vi "Decode Reply.vi"(5 "ProcessID":u32 format="%04x", 6 "RxTimeStamp":u32, 7 "TxTimeStamp Alt":u32, 10 "ICMP Packet Info":T3 {"Sequence Number" format="%04x"; "ID" format="%04x"; "Checksum" format="%04x"; "Data" format="%02x"}, 11 "IP Packet":T2 {"Header Checksum" format="%04x"; "Flags" format="%02x"; "Type of Service" format="%02x"}) -> (0 "Error Out":errorcluster, 1 "Done?":bool, 3 "Ping Reply Info":T1 {"Sequence" format="%04x"})   [LabVIEW 2018]
uses:
  ICMP Packet Info.ctl
  IP Packet Info.ctl
  Ping Reply Info.ctl
  Instance           2 20Saved   Decode Reply .vi
  Instance           1 20Saved   Decode Reply .vi
panel:
  in  "Error In":errorcluster
  # "Use the process ID we obtained when sending the ping to make sure we have received the correct reply"
  # "The tick count is encoded in the ping packet, but if we want to try and make\na time measurement more accurate we can use a time stamp taken when\nthe packet is sent, not when it is encoded.  This deprives us of being able\nto send a bunch of pings at the same time and calculate arrival time back,\nbut that's ok in most circumstances."
  # "U8"
  # "U8"
  # "U16"
  # "U16"
  # "U16"
  # "U32"
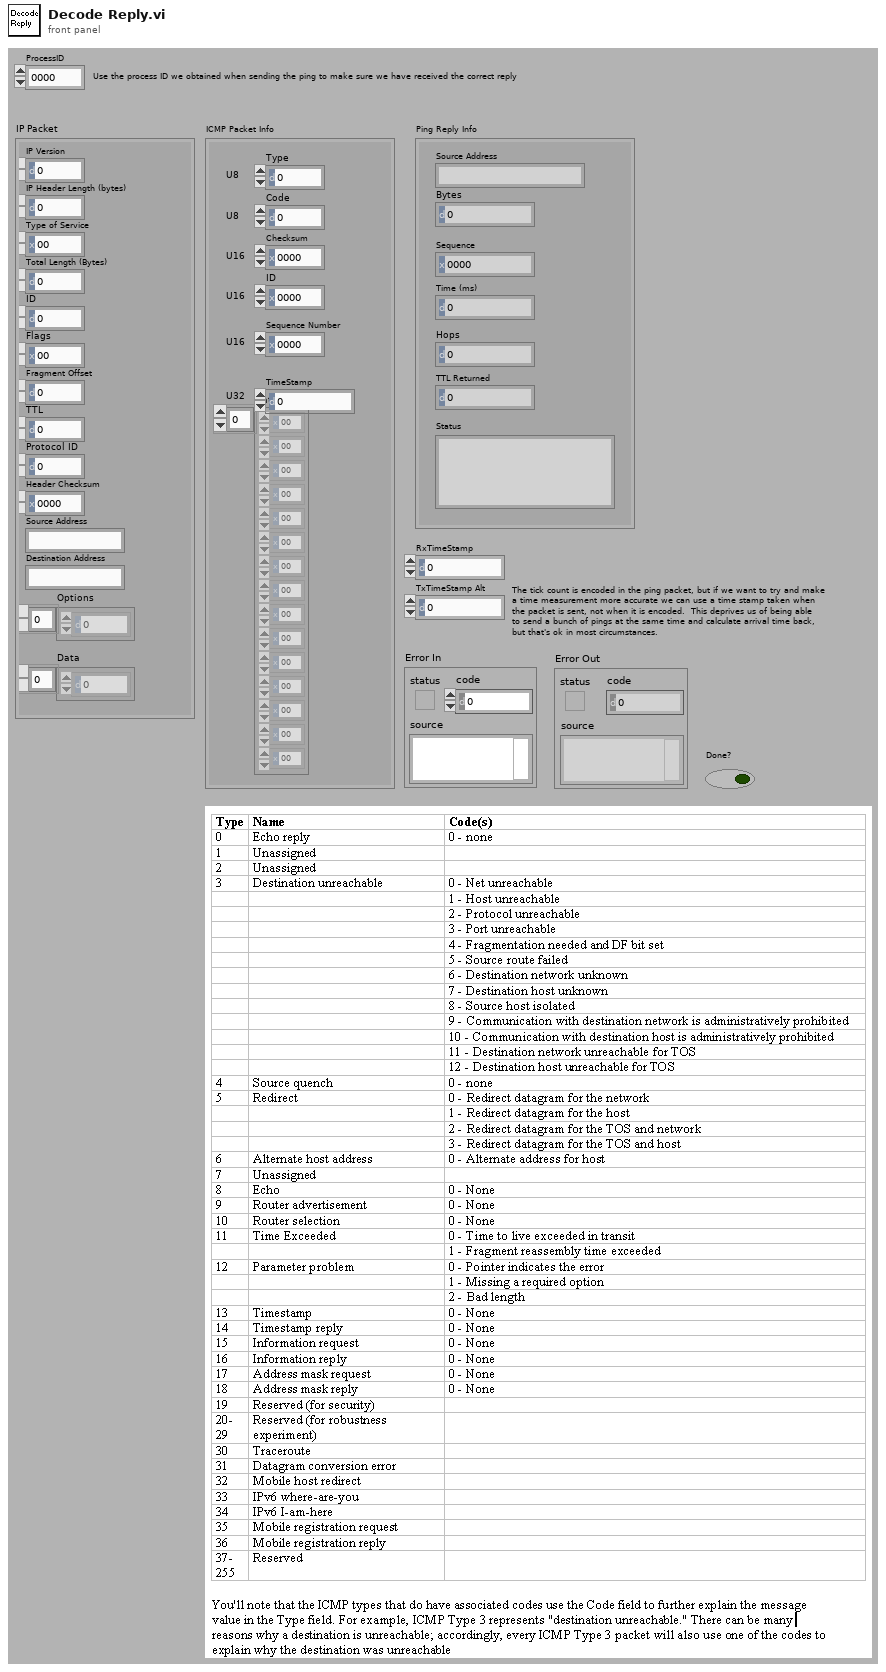
[diagram p1: front panel]
types:
  T1 = typedef "Ping Reply Info.ctl" = cluster{"Source Address":string, "Bytes":i32, "Sequence":u16, "Time (ms)":i32, "Hops":u8, "TTL Returned":u8, "Status":string}
  T2 = typedef "IP Packet Info.ctl" = cluster{"IP Version":u8, "IP Header Length (bytes)":u8, "Type of Service":u8, "ID":u16, "Flags":u8, "Total Length (Bytes)":u16, "Fragment Offset":u16, "TTL":u8, "Protocol ID":u8, "Header Checksum":u16, "Source Address":string, "Destination Address":string, "Options":u8[], "Data":u8[]}
  T3 = typedef "ICMP Packet Info.ctl" = cluster{"Type":u8, "Code":u8, "Checksum":u16, "ID":u16, "Sequence Number":u16, "TimeStamp":u32, "Data":u8[]}
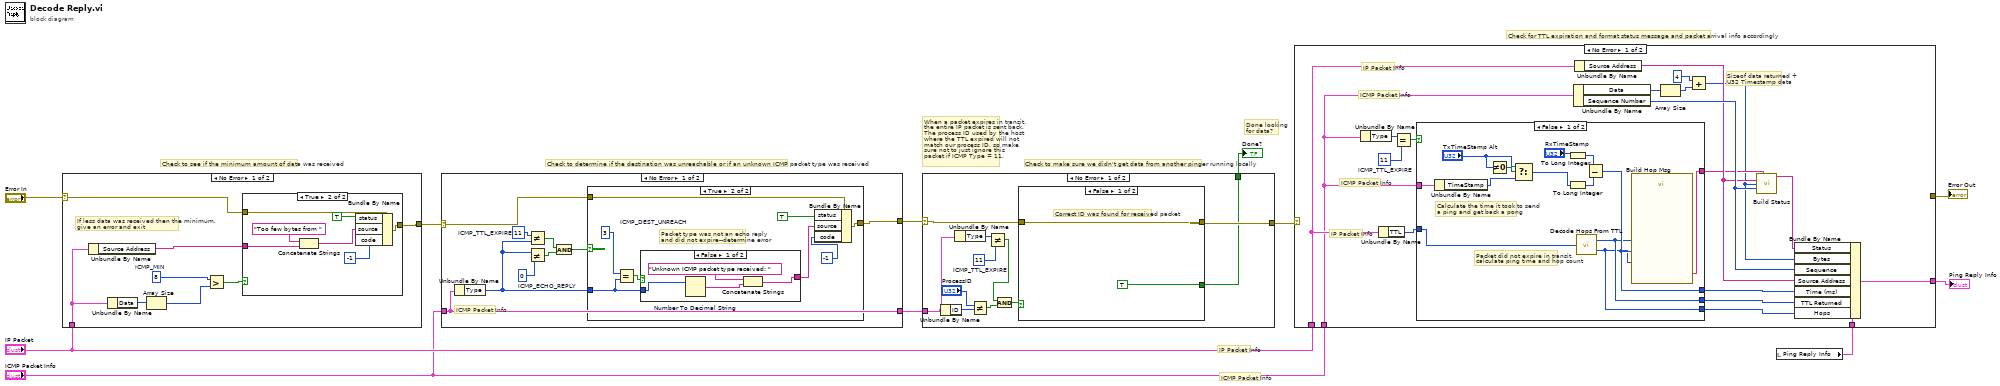
[diagram p0: block diagram]
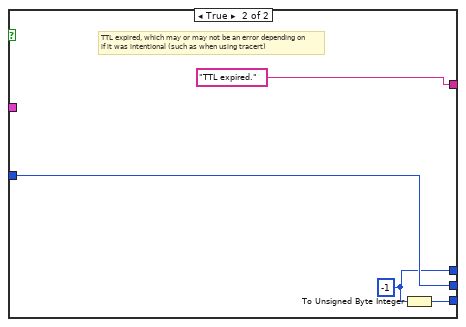
[diagram p2: hidden frame]
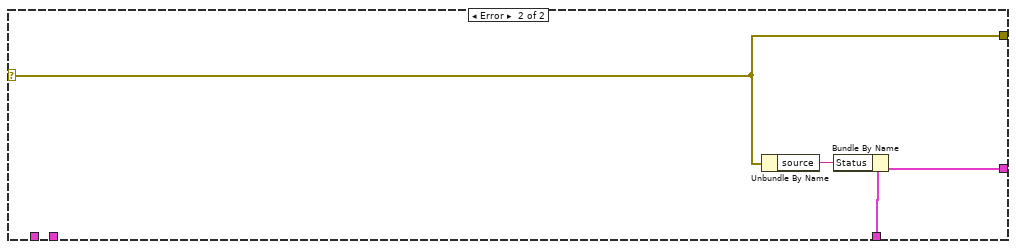
[diagram p3: hidden frame]
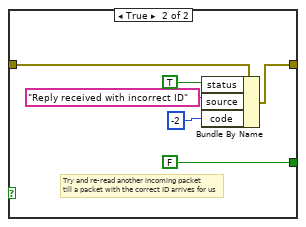
[diagram p4: hidden frame]
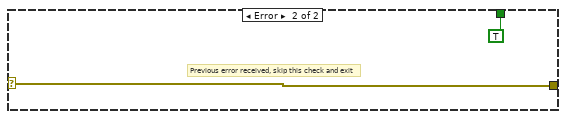
[diagram p5: hidden frame]
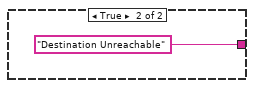
[diagram p7: hidden frame]
diagram:
  # "Done looking\nfor data?"
  # "When a packet expires in transit,\nthe entire IP packet is sent back.\nThe process ID used by the host\nwhere the TTL expired will not\nmatch our process ID, so make\nsure not to just ignore this \npacket if ICMP Type = 11."
  # "Check for TTL expiration and format status message and packet arrival info accordingly"
  # "ICMP Packet Info"
  # "IP Packet Info"
  # "Check to make sure we didn't get data from another pinger running locally"
  # "Check to determine if the destination was unreachable or if an unknown ICMP packet type was received"
  # "Check to see if the minimum amount of data was received"
  n1 = case shown="No Error" "Error In" {
    selector: "Error In" -> [w18 w28]
    tunnel: [w17 w28] -> w10
    tunnel: "IP Packet" -> [w16 _]
    frame No Error {
      w12 = u8 8  # ICMP_MIN
      # "If less data was received then the minimum,\ngive an error and exit"
      n2 = Unbundle By Name(w16) -> ("Source Address"=w19:string)
      n3 = Unbundle By Name(w16) -> ("Data"=w15:u8[])
      n4 = Array Size(array=w15) -> (size(s)=w14:i32)
      n5 = Greater?(x=w12, y=w14) -> (0:w13:bool)
      n6 = case shown="True" w13 {
        tunnel: w19 -> [_ w27]
        tunnel: w18 -> [w20 w26]
        tunnel: [w20 w23] -> w17
        frame False {
        }
        frame True {
          n7 = Concatenate Strings("Too few bytes from ", w27) -> (w25:string)
          n8 = Bundle By Name(cluster=w26, "status"=TRUE, "source"=w25, "code"=-1) -> (w23:errorcluster)
        }
      }
    }
    frame Error {
    }
  }
  n9 = case shown="No Error" w10 {
    selector: w10 -> [w37 w52]
    tunnel: [w30 w52] -> w8
    tunnel: "ICMP Packet Info" -> [w29 _]
    tunnel: [w29 _] -> w9
    frame No Error {
      w33 = u8 11  # ICMP_TTL_EXPIRE
      w36 = u8 0  # ICMP_ECHO_REPLY
      # "ICMP Packet Info"
      n10 = Unbundle By Name(w29) -> ("Type"=w31:u8)
      n11 = Not Equal?(x=w33, y=w31) -> (x != y?=w34:bool)
      n12 = Not Equal?(x=w31, y=w36) -> (x != y?=w35:bool)
      n13 = Compound Arithmetic op=AND(w34, w35) -> (w32:bool)
      n14 = case shown="True" w32 {
        tunnel: w37 -> [w38 w45]
        tunnel: [w38 w39] -> w30
        tunnel: w31 -> [_ w41]
        frame False {
          # "Echo Reply was received, or TTL expired,\neither way press on,\nTTL expiration checked sequentially after\nthis so the error will not be missed"
        }
        frame True {
          w46 = u8 3  # ICMP_DEST_UNREACH
          # "Packet type was not an echo reply\nand did not expire--determine error"
          n15 = Equal?(x=w46, y=w41) -> (x = y?=w43:bool)
          n16 = case shown="False" w43 {
            tunnel: [w47 "Destination Unreachable"] -> w42
            tunnel: w41 -> [w50 _]
            frame False {
              n17 = Number To Decimal String(number=w50) -> (decimal integer string=w49:string)  [unwired: 1 in]
              n18 = Concatenate Strings("Unknown ICMP packet type received: ", w49) -> (w47:string)
            }
            frame True {
            }
          }
          n19 = Bundle By Name(cluster=w45, "status"=TRUE, "source"=w42, "code"=-1) -> (w39:errorcluster)
        }
      }
    }
    frame Error {
      # "Previous error received, skip this check and exit"
    }
  }
  n20 = case shown="No Error" w8 {
    selector: w8 -> [w61 w73]
    tunnel: w9 -> [w54 _]
    tunnel: [w60 w73] -> w7
    tunnel: [w53 TRUE ("status")] -> w1
    frame No Error {
      w57 = u8 11  # ICMP_TTL_EXPIRE
      n21 = Unbundle By Name(w54) -> ("ID"=w63:u16)
      n22 = Unbundle By Name(w54) -> ("Type"=w56:u8)
      n23 = Not Equal?(x="ProcessID", y=w63) -> (x != y?=w59:bool)
      n24 = Not Equal?(x=w56, y=w57) -> (x != y?=w55:bool)
      n25 = Compound Arithmetic op=AND(w55, w59) -> (w58:bool)
      n26 = case shown="False" w58 {
        tunnel: w61 -> [w65 w71]
        tunnel: [w65 w67] -> w60
        tunnel: [TRUE ("status") FALSE ("status")] -> w53
        frame False {
          # "Correct ID was found for received packet"
        }
        frame True {
          # "Try and re-read another incoming packet\ntill a packet with the correct ID arrives for us"
          n27 = Bundle By Name(cluster=w71, "status"=TRUE, "source"="Reply received with incorrect ID", "code"=-2) -> (w67:errorcluster)
        }
      }
    }
    frame Error {
      # "Previous error received, skip this check and exit"
    }
  }
  "Done?" <- w1
  n28 = local read "Ping Reply Info"() -> (w2:T1)
  n29 = case shown="No Error" w7 {
    selector: w7 -> [_ w111]
    tunnel: "IP Packet" -> [w80 _]
    tunnel: "ICMP Packet Info" -> [w79 _]
    tunnel: [_ w111] -> w5
    tunnel: [w75 w113] -> w3
    tunnel: w2 -> [w74 w112]
    frame No Error {
      w81 = u8 11  # ICMP_TTL_EXPIRE
      # "IP Packet Info"
      # "IP Packet Info"
      # "ICMP Packet Info"
      # "ICMP Packet Info"
      # "Sizeof data returned + \nU32 Timestamp data"
      n30 = Unbundle By Name(w79) -> ("Type"=w82:u8)
      n31 = Unbundle By Name(w80) -> ("TTL"=w89:u8)
      n32 = Equal?(x=w82, y=w81) -> (x = y?=w84:bool)
      n33 = case shown="False" w84 {
        tunnel: [w105 "TTL expired."] -> w85
        tunnel: w79 -> [w101 _]
        tunnel: [w100 w108] -> w86
        tunnel: [w94 w109] -> w87
        tunnel: [w93 w107] -> w88
        tunnel: w89 -> [w95 w109]
        frame False {
          # "Packet did not expire in transit,\ncalculate ping time and hop count"
          # "Calculate the time it took to send \na ping and get back a pong"
          n34 = Unbundle By Name(w101) -> ("TimeStamp"=w99:u32)
          n35 = Not Equal To 0?(x="TxTimeStamp Alt") -> (x != 0?=w97:bool)
          n36 = Select(t="TxTimeStamp Alt", s=w97, f=w99) -> (s? t:f=w98:u32)
          n37 = To Long Integer(number="RxTimeStamp") -> (32bit integer=w103:i32)
          n38 = To Long Integer(number=w98) -> (32bit integer=w102:i32)
          n39 = call "Decode Hops From TTL.vi"("TTL"=w95) -> ("TTL Out"=w94:u8, "Hops"=w93:u8)
          n40 = Subtract(x=w103, y=w102) -> (x-y=w100:i32)
          n41 = call "Build Hop Msg"("TimeDifference (ms)"=w100, "TTL"=w94, "Hops"=w93) -> ("Result"=w105:string)  [unwired: 11 in, 1 out]
        }
        frame True {
          w108 = -1
          # "TTL expired, which may or may not be an error depending on\nif it was intentional (such as when using tracert)"
          n42 = To Unsigned Byte Integer(number=w108) -> (unsigned 8bit integer=w107:u8)
        }
      }
      n43 = Unbundle By Name(w79) -> ("Data"=w83:u8[], "Sequence Number"=w91:u16)
      n44 = Unbundle By Name(w80) -> ("Source Address"=w90:string)
      n45 = Array Size(array=w83) -> (size(s)=w78:i32)
      n46 = Add(x=4, y=w78) -> (x+y=w76:i32)
      n47 = call "Build Status"("Hop/Expiration Msg"=w85, "IP"=w90, "Bytes Read"=w76, "Sequence"=w91) -> ("Result"=w92:string)  [unwired: 10 in, 1 out]
      n48 = Bundle By Name(cluster=w74, "Status"=w92, "Bytes"=w76, "Sequence"=w91, "Source Address"=w90, "Time (ms)"=w86, "TTL Returned"=w87, "Hops"=w88) -> (w75:T1)
    }
    frame Error {
      n49 = Unbundle By Name(w111) -> ("source"=w110:string)
      n50 = Bundle By Name(cluster=w112, "Status"=w110) -> (w113:T1)
    }
  }
  "Error Out" <- w5
  "Ping Reply Info" <- w3
